vi "loop_test.vi"() -> ()   [LabVIEW 2021]
panel:
  out "out":dbl
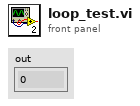
[diagram p1: front panel]
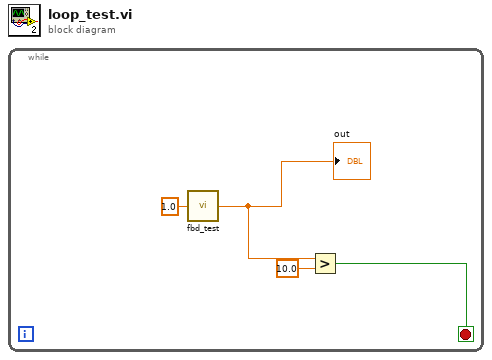
[diagram p0: block diagram]
diagram:
  n1 = while {
    stop <- w1 stop-if-true
    n2 = call "fbd_test.vi"("in"=1.0) -> ("out"=w3:dbl)
    "out" <- w3
    n3 = Greater?(x=w3, y=10.0) -> (0:w1:bool)
  }
